vi "DAQ_pp3d_stateToMaster9Int.vi"(11 "State In":T1={"Curr  tr"=0, "Curr (ms)"=0, "Cum (ms)"=0, "Run loop diff"=0, "Tone countdown (ms)"=0, "Countdown (ms)"=0, "Curr State"=enum."0 NULL", "Prev State"=enum."0 NULL", "Rw"=FALSE, "Sw"=FALSE, "Tone\nGate"=FALSE, "Punish"=FALSE, "Current DAQ DO Int"=0, "Current Loaded Trial"={"Trial Type Number"=1, "Trial Type"=enum."GO", "Trial Weight"=100, "Shock (mA)"=0.3, "Duration (ms)"=0.25, "Sound Type"=enum."04 FM Sweep", "Stim P1"=4000.0, "Stim P2"=0.0, "Stim P3"=0.0, "Stim P4"=2000.0, "DAQ Amplitude (V)"=0.25}, "Total trials memo"=0, "State start cum memo (ms)"=0, "Last dur jump time memo (ms)"=0, "Last dur shock time memo (ms)"=0, "Tone repeat memo (ms)"=0, "Webcam on"=FALSE, "Webcam recording"=FALSE, "State update flag"=FALSE, "Last loaded shock voltage"=0.0, "Vid upd"=enum."0", "First time tone"=FALSE} {"Current DAQ DO Int" format="%016b"; "Current Loaded Trial"."DAQ Amplitude (V)" min=0.0 max=5.0 format="%_4g"; "Current Loaded Trial"."Shock (mA)" min=-1.0 max=5.0; "Current Loaded Trial"."Trial Weight" step=1; "Current Loaded Trial"."Duration (ms)" min=0.0 max=1.0; "Current Loaded Trial"."Trial Type Number" min=1 max=256 step=1}) -> (3 "Master-9 Output Array":bool[](array[boolean]))   [LabVIEW 2013]
uses:
  CTL_pp3g_LoopState.ctl
  pp3_CTL_BehavioralState.ctl
  CTL_pp3g_Trial.ctl
  pp3_CTL_TrialType.ctl
  labolabo2/waveforms/WFTypes.ctl
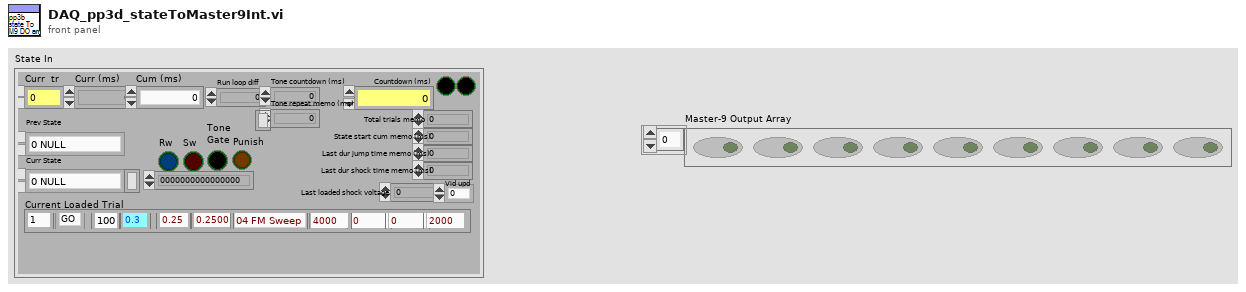
[diagram p1: front panel]
types:
  T1 = typedef "CTL_pp3g_LoopState.ctl" = cluster{"Curr  tr":u16, "Curr (ms)":u32, "Cum (ms)":u64, "Run loop diff":i64, "Tone countdown (ms)":i64, "Countdown (ms)":i64, "Curr State":T2, "Prev State":T2, "Rw":bool, "Sw":bool, "Tone\nGate":bool, "Punish":bool, "Current DAQ DO Int":u16, "Current Loaded Trial":T3, "Total trials memo":i64, "State start cum memo (ms)":i64, "Last dur jump time memo (ms)":i64, "Last dur shock time memo (ms)":i64, "Tone repeat memo (ms)":i64, "Webcam on":bool, "Webcam recording":bool, "State update flag":bool, "Last loaded shock voltage":dbl, "Vid upd":enum16{"0", "1", "2", "3", "4", "5", "6", "7", "8", "9"}, "First time tone":bool}
  T2 = typedef "pp3_CTL_BehavioralState.ctl" = enum8{"0 NULL", "1 Habituation", "2 (Load Trial)", "3 Stay Period", "4 Load Audio/Click Delay", "5 GO Trial", "6 GO Jumped", "7 GO Timeout", "8 NOGO Trial", "9 NOGO Jumped", "10 NOGO Timeout", "11 TEST Trial", "12 TEST Jumped", "13 TEST Timeout", "14 Intertrial Interval", "15 Done"}
  T3 = typedef "CTL_pp3g_Trial.ctl" = cluster{"Trial Type Number":i16, "Trial Type":T4, "Trial Weight":u32, "Shock (mA)":dbl, "Duration (ms)":dbl, "Sound Type":T5, "Stim P1":dbl, "Stim P2":dbl, "Stim P3":dbl, "Stim P4":dbl, "DAQ Amplitude (V)":dbl}
  T4 = typedef "pp3_CTL_TrialType.ctl" = enum16{"OFF", "GO", "NOGO", "TEST"}
  T5 = typedef "WFTypes.ctl" = enum16{"00 NULL", "01 DC", "02 Noise", "03 Pure Tone", "04 FM Sweep", "05 FM Sweep BURST"}
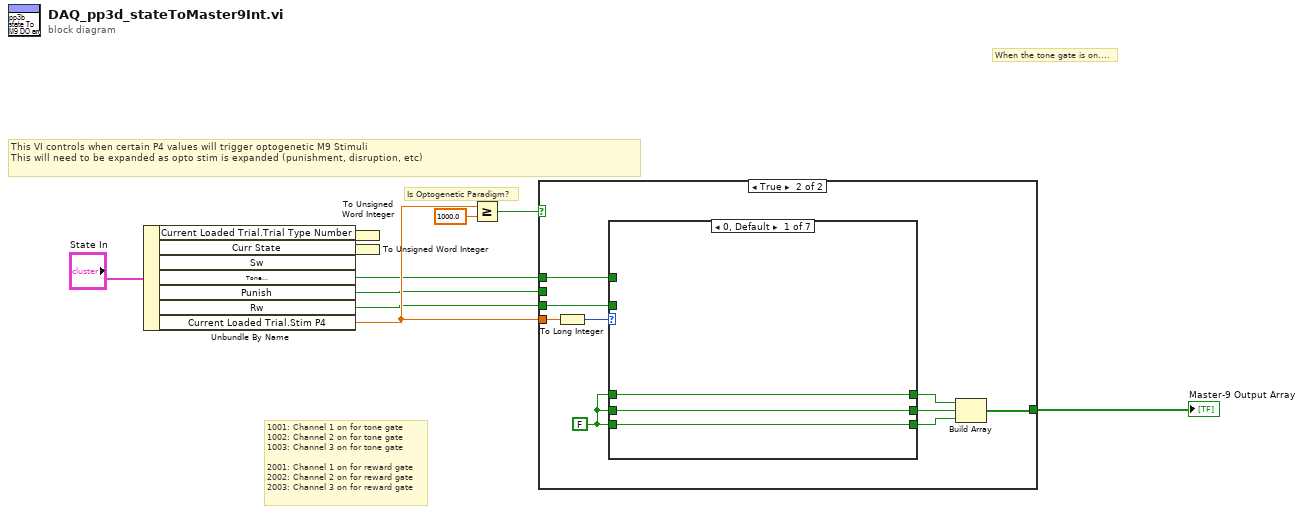
[diagram p0: block diagram]
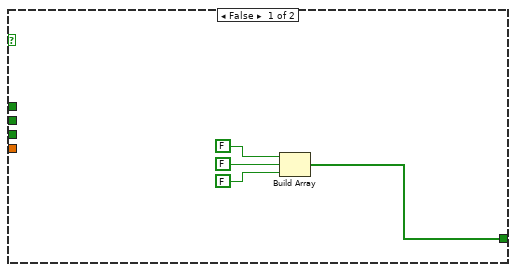
[diagram p2: hidden frame]
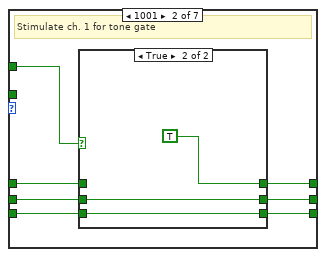
[diagram p3: hidden frame]
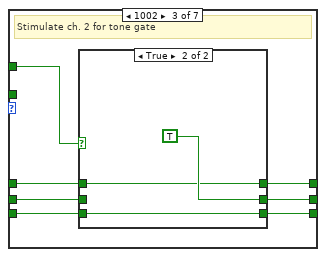
[diagram p5: hidden frame]
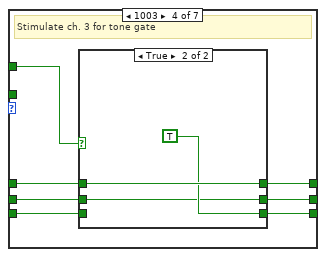
[diagram p7: hidden frame]
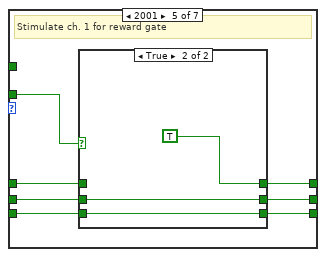
[diagram p9: hidden frame]
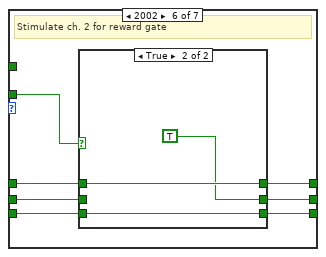
[diagram p11: hidden frame]
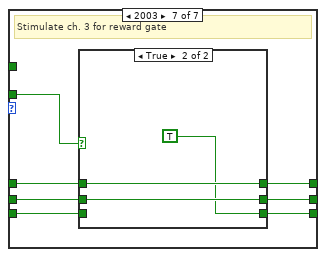
[diagram p13: hidden frame]
diagram:
  # "1001: Channel 1 on for tone gate\n1002: Channel 2 on for tone gate\n1003: Channel 3 on for tone gate\n\n2001: Channel 1 on for reward gate\n2002: Channel 2 on for reward gate\n2003: Channel 3 on for reward gate"
  # "Is Optogenetic Paradigm?"
  # "When the tone gate is on...."
  # "This VI controls when certain P4 values will trigger optogenetic M9 Stimuli\nThis will need to be expanded as opto stim is expanded (punishment, disruption, etc)"
  n1 = Unbundle By Name("State In") -> ("Current Loaded Trial.Trial Type Number"=w9:i16, "Curr State"=w8:T2, "Tone\nGate"=w4:bool, "Punish"=w3:bool, "Rw"=w2:bool, "Current Loaded Trial.Stim P4"=w5:dbl)  [unwired: 1 out]
  n2 = To Unsigned Word Integer(number=w9) -> ()  [unwired: 1 out]
  n3 = To Unsigned Word Integer(number=w8) -> ()  [unwired: 1 out]
  n4 = Greater Or Equal?(x=w5, y=1000.0) -> (x >= y?=w6:bool)
  n5 = case shown="True" w6 {
    tunnel: w5 -> [_ w22]
    tunnel: w4 -> [_ w16]
    tunnel: w3 -> [_ _]
    tunnel: w2 -> [_ w15]
    tunnel: [w11 w21] -> w1
    frame False {
      n6 = Build Array(FALSE, FALSE, FALSE) -> (w11:bool[])
    }
    frame True {
      w17 = FALSE
      n7 = To Long Integer(number=w22) -> (32bit integer=w23:i32)
      n8 = case shown="0, Default" w23 {
        tunnel: [w26 w33 w46 w59 w72 w85 w98] -> w20
        tunnel: [w25 w31 w44 w57 w71 w84 w97] -> w19
        tunnel: [w24 w29 w42 w55 w69 w82 w95] -> w18
        tunnel: w17 -> [w24 w28 w41 w54 w68 w81 w94]
        tunnel: w17 -> [w25 w30 w43 w56 w70 w83 w96]
        tunnel: w17 -> [w26 w27 w40 w53 w67 w80 w93]
        tunnel: w16 -> [_ w32 w45 w58 _ _ _]
        tunnel: w15 -> [_ _ _ _ w66 w79 w92]
        frame 0, Default {
        }
        frame 1001 {
          # "Stimulate ch. 1 for tone gate"
          n9 = case shown="True" w32 {
            tunnel: [w36 TRUE] -> w33
            tunnel: [w35 w38] -> w31
            tunnel: w30 -> [w35 w38]
            tunnel: [w34 w37] -> w29
            tunnel: w28 -> [w34 w37]
            tunnel: w27 -> [w36 _]
            frame False {
            }
            frame True {
            }
          }
        }
        frame 1002 {
          # "Stimulate ch. 2 for tone gate"
          n10 = case shown="True" w45 {
            tunnel: [w49 w50] -> w46
            tunnel: [w48 TRUE] -> w44
            tunnel: w43 -> [w48 _]
            tunnel: [w47 w52] -> w42
            tunnel: w41 -> [w47 w52]
            tunnel: w40 -> [w49 w50]
            frame False {
            }
            frame True {
            }
          }
        }
        frame 1003 {
          # "Stimulate ch. 3 for tone gate"
          n11 = case shown="True" w58 {
            tunnel: [w62 w65] -> w59
            tunnel: [w61 w63] -> w57
            tunnel: w56 -> [w61 w63]
            tunnel: [w60 TRUE] -> w55
            tunnel: w54 -> [w60 _]
            tunnel: w53 -> [w62 w65]
            frame False {
            }
            frame True {
            }
          }
        }
        frame 2001 {
          # "Stimulate ch. 1 for reward gate"
          n12 = case shown="True" w66 {
            tunnel: [w75 TRUE] -> w72
            tunnel: [w74 w78] -> w71
            tunnel: w70 -> [w74 w78]
            tunnel: [w73 w77] -> w69
            tunnel: w68 -> [w73 w77]
            tunnel: w67 -> [w75 _]
            frame False {
            }
            frame True {
            }
          }
        }
        frame 2002 {
          # "Stimulate ch. 2 for reward gate"
          n13 = case shown="True" w79 {
            tunnel: [w88 w90] -> w85
            tunnel: [w87 TRUE] -> w84
            tunnel: w83 -> [w87 _]
            tunnel: [w86 w91] -> w82
            tunnel: w81 -> [w86 w91]
            tunnel: w80 -> [w88 w90]
            frame False {
            }
            frame True {
            }
          }
        }
        frame 2003 {
          # "Stimulate ch. 3 for reward gate"
          n14 = case shown="True" w92 {
            tunnel: [w101 w104] -> w98
            tunnel: [w100 w103] -> w97
            tunnel: w96 -> [w100 w103]
            tunnel: [w99 TRUE] -> w95
            tunnel: w94 -> [w99 _]
            tunnel: w93 -> [w101 w104]
            frame False {
            }
            frame True {
            }
          }
        }
      }
      n15 = Build Array(w20, w19, w18) -> (w21:bool[])
    }
  }
  "Master-9 Output Array" <- w1
